vi "Write Value (variant).vi"(8 "error in (no error)":errorcluster, 10 "Variant":variant, 11 "Ring D Element in":refnum<class "String dropdown D Element.lvclass">) -> (0 "error out":errorcluster, 3 "Ring D Element out":refnum<class "String dropdown D Element.lvclass">)   [LabVIEW 2018, in "D Datagrid Library.lvlib" / "String dropdown D Element.lvclass"]
uses:
  String dropdown D Element.lvclass
  String dropdown D Element.lvclass/String dropdown D Element.ctl
  Write value.vi
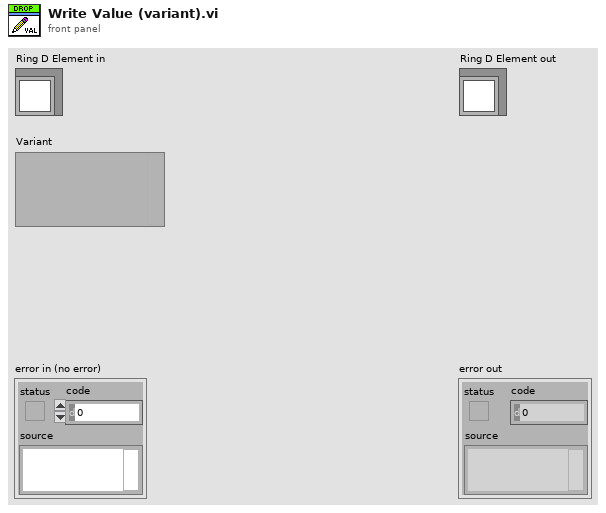
[diagram p1: front panel]
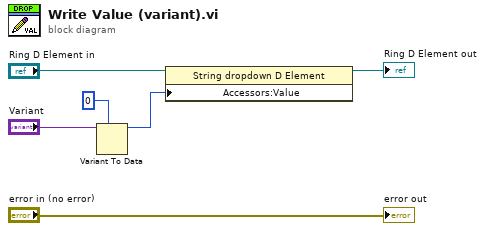
[diagram p0: block diagram]
diagram:
  n1 = Variant To Data(type=0 ("Selected index"), Variant="Variant") -> (data=w1:i32)  [unwired: 1 in, 1 out]
  n2 = property class="String dropdown D Element"(reference="Ring D Element in", "Accessors:Value"=w1) -> (reference out=→"Ring D Element out":refnum<class "String dropdown D Element.lvclass">)  [unwired: 1 in, 1 out]
  "error out" <- "error in (no error)"
